vi "SeCrTs-DI_Scale_Config.vi"(8 "error in (no error)":errorcluster, 10 "DI config":T1(array[cluster]), 11 "Refnum in":refnum<k21>) -> (0 "error out":errorcluster, 3 "Refnum out":refnum<k21>)   [LabVIEW 2022 SP3]
uses:
  <vilib>/DAQmx/create/channels.llb/DAQmx Create Channel (DI-Digital Input).vi
  <resource>/objmgr/daqmx.rc
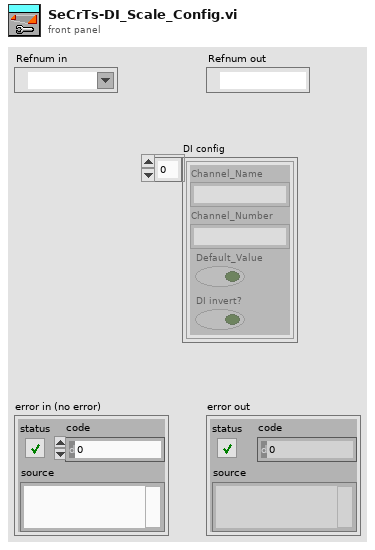
[diagram p1: front panel]
types:
  T1 = cluster{"Channel_Name":string, "Channel_Number":string, "Default_Value":bool, "DI invert?":bool}[]
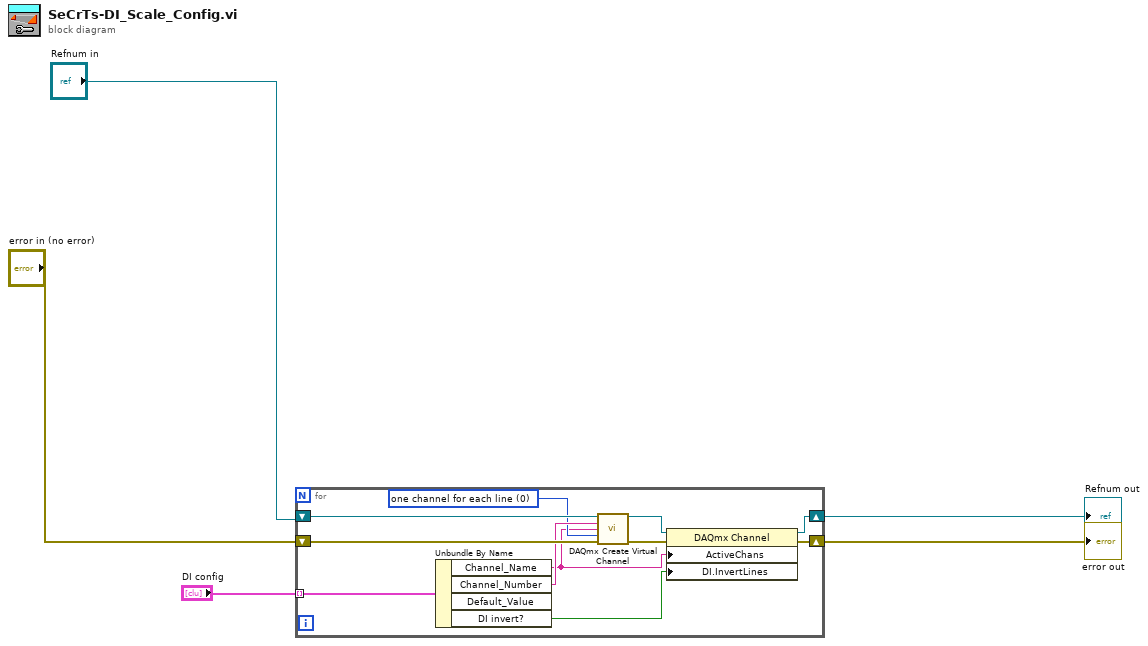
[diagram p0: block diagram]
diagram:
  n1 = for {
    tunnel: "DI config" -> [w16] mode=indexing
    shift-right: [w9] -> w2
    shift-left: "Refnum in" -> [w15]
    shift-right: [w8] -> w3
    shift-left: "error in (no error)" -> [w14]
    w12 = 0 items=["one channel for each line", "one channel for all lines"] ("line grouping")
    n2 = Unbundle By Name(w16) -> ("Channel_Name"=w7:string, "Channel_Number"=w13:string, "DI invert?"=w6:bool)  [unwired: 1 out]
    n3 = call-poly <vilib>:"DAQmx Create Virtual Channel.vi"("task in"=w15, "lines"=w13, "name to assign"=w7, "line grouping"=w12, "error in"=w14) -> ("task out"=w11:refnum<k21>, "error out"=w10:errorcluster)  [unwired: 9 in]
    n4 = property on="Property Node" class="DAQmx Channel"(reference=w11, error in=w10, "ActiveChans"=w7, "DI.InvertLines"=w6) -> (reference out=w9:refnum<k21>, error out=w8:errorcluster)
  }
  "error out" <- w3
  "Refnum out" <- w2
